vi "record selected tracks.vi"(6 "index":i32, 7 "Track Controls":T1 {"Track 3"."Volume Settings"."Volume" scale=1.0..10.0; "Track 3"."Volume Settings"."Pan" scale=0.0..1.0; "Track 3"."Effects Settings"."Delay 2" scale=0.0..10.0; "Track 3"."Effects Settings"."Delay" scale=0.0..1.0; "Track 2"."Volume Settings"."Volume" scale=1.0..10.0; "Track 2"."Volume Settings"."Pan" scale=0.0..1.0; "Track 2"."Effects Settings"."Delay 2" scale=0.0..10.0; "Track 2"."Effects Settings"."Delay" scale=0.0..1.0; "Track 1"."Volume Settings"."Volume" scale=1.0..10.0; "Track 1"."Volume Settings"."Pan" scale=0.0..1.0; "Track 1"."Effects Settings"."Delay 2" scale=0.0..10.0; "Track 1"."Effects Settings"."Delay" scale=0.0..1.0; "Track 0"."Volume Settings"."Volume" scale=1.0..10.0; "Track 0"."Volume Settings"."Pan" scale=0.0..1.0; "Track 0"."Effects Settings"."Delay 2" scale=0.0..10.0; "Track 0"."Effects Settings"."Delay" scale=0.0..1.0}, 9 "AudioIn/Right (N Samples)":i16[](array[numeric]), 10 "AudioIn/Left (N Samples)":i16[](array[numeric]), 11 "4-Track Audio in":T5) -> (3 "4-Track Audio out":T5)   [LabVIEW 2014]
uses:
  Controls/4 Track Audio.ctl
  Controls/Audio In.ctl
  Controls/Track Controls.ctl
  Controls/Track Settings.ctl
  Controls/Track Effects Settings.ctl
  Controls/Track Volume Settings.ctl
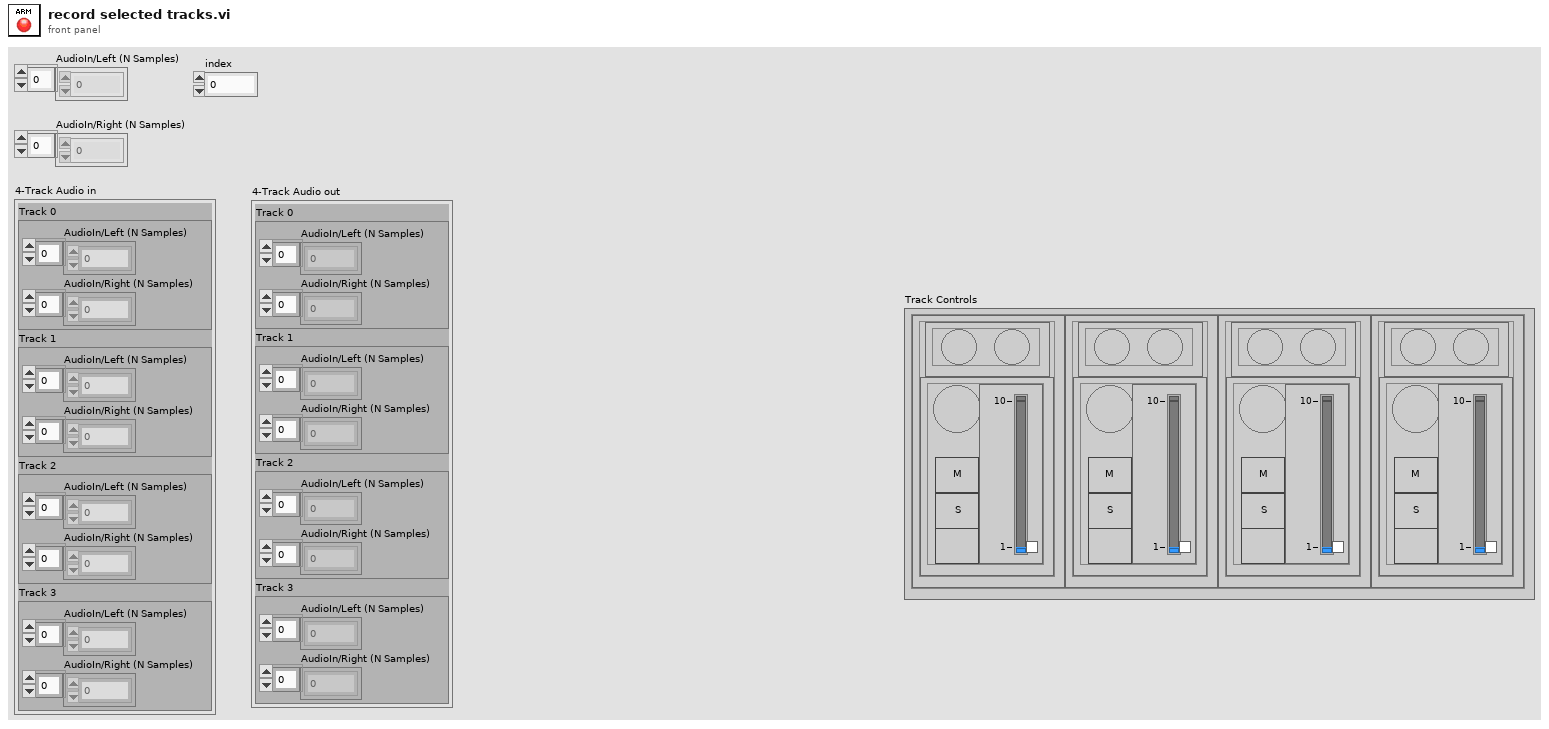
[diagram p1: front panel]
types:
  T1 = typedef "Track Controls.ctl" = cluster{"Track 0":T2, "Track 1":T2, "Track 2":T2, "Track 3":T2}
  T2 = typedef "Track Settings.ctl" = cluster{"Effects Settings":T3, "Volume Settings":T4}
  T3 = typedef "Track Effects Settings.ctl" = cluster{"Delay":dbl, "Delay 2":dbl}
  T4 = typedef "Track Volume Settings.ctl" = cluster{"Mute":bool, "Solo":bool, "Record":bool, "Pan":dbl, "Volume":dbl}
  T5 = typedef "4 Track Audio.ctl" = cluster{"Track 0":T6, "Track 1":T6, "Track 2":T6, "Track 3":T6}
  T6 = typedef "Audio In.ctl" = cluster{"AudioIn/Left (N Samples)":i16[], "AudioIn/Right (N Samples)":i16[]}
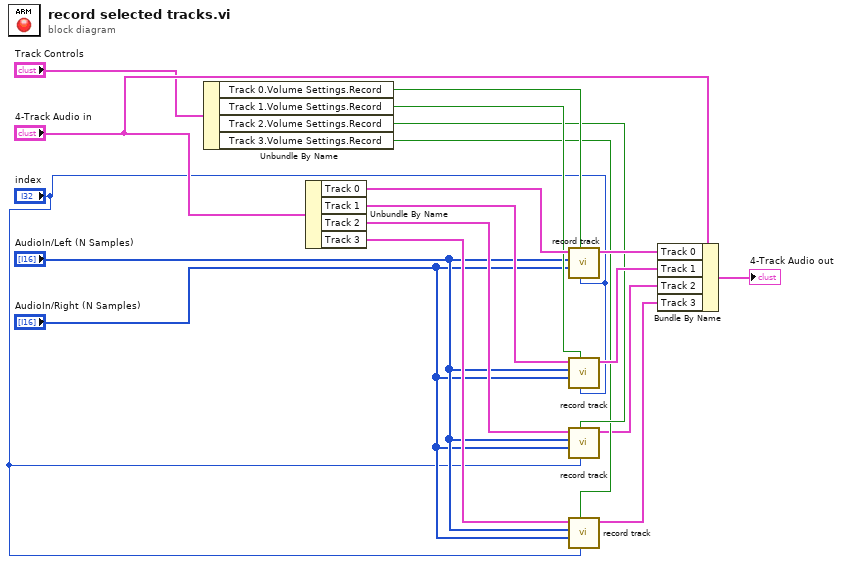
[diagram p0: block diagram]
diagram:
  n1 = Unbundle By Name("Track Controls") -> ("Track 0.Volume Settings.Record"=w14:bool, "Track 1.Volume Settings.Record"=w12:bool, "Track 2.Volume Settings.Record"=w9:bool, "Track 3.Volume Settings.Record"=w7:bool)
  n2 = Unbundle By Name("4-Track Audio in") -> ("Track 0"=w13:T6, "Track 1"=w11:T6, "Track 2"=w8:T6, "Track 3"=w6:T6)
  n3 = call "record track.vi"("index"="index", "Record"=w14, "AudioIn/Right (N Samples)"="AudioIn/Right (N Samples)", "AudioIn/Left (N Samples)"="AudioIn/Left (N Samples)", "Track In"=w13) -> ("Track Out"=w15:T6)  [unwired: 6 in]
  n4 = call "record track.vi"("index"="index", "Record"=w12, "AudioIn/Right (N Samples)"="AudioIn/Right (N Samples)", "AudioIn/Left (N Samples)"="AudioIn/Left (N Samples)", "Track In"=w11) -> ("Track Out"=w10:T6)  [unwired: 6 in]
  n5 = call "record track.vi"("index"="index", "Record"=w9, "AudioIn/Right (N Samples)"="AudioIn/Right (N Samples)", "AudioIn/Left (N Samples)"="AudioIn/Left (N Samples)", "Track In"=w8) -> ("Track Out"=w5:T6)  [unwired: 6 in]
  n6 = call "record track.vi"("index"="index", "Record"=w7, "AudioIn/Right (N Samples)"="AudioIn/Right (N Samples)", "AudioIn/Left (N Samples)"="AudioIn/Left (N Samples)", "Track In"=w6) -> ("Track Out"=w4:T6)  [unwired: 6 in]
  n7 = Bundle By Name(cluster="4-Track Audio in", "Track 0"=w15, "Track 1"=w10, "Track 2"=w5, "Track 3"=w4) -> (→"4-Track Audio out":T5)
